vi "PicoCmdClientMove_5.vi"(1 "APulsesButton":bool, 2 "DeviceID":T1, 3 "Error in":errorcluster, 4 "ARateButton":bool, 5 "APulses":u16=300 step=100, 6 "Reverse":cluster{"Reverse X":bool, "Reverse Y":bool}, 7 "AXIS":u16(ring) items=["X", "Y or SLIDE", "Z"], 8 "aRate":dbl(ring)=1500.0 items=["375Hz"=375.0, "500Hz"=500.0, "750Hz"=750.0, "1500Hz"=1500.0], 9 "Move XY":T2(array[cluster]), 11 "aDir":bool=TRUE, 12 "connection ID in":refnum<k5>, 13 "aStop":bool, 16 "client name":string, 17 "Response?":bool) -> (20 "connection ID out":refnum<k5>, 21 "TCPconnectionCmd":bool, 25 "status":string, 27 "error out":errorcluster)   [LabVIEW 2013]
panel:
  out "Port":i32
  out "IPaddress":string
  out "mirror SlotConnector":i32
  out "Command":string
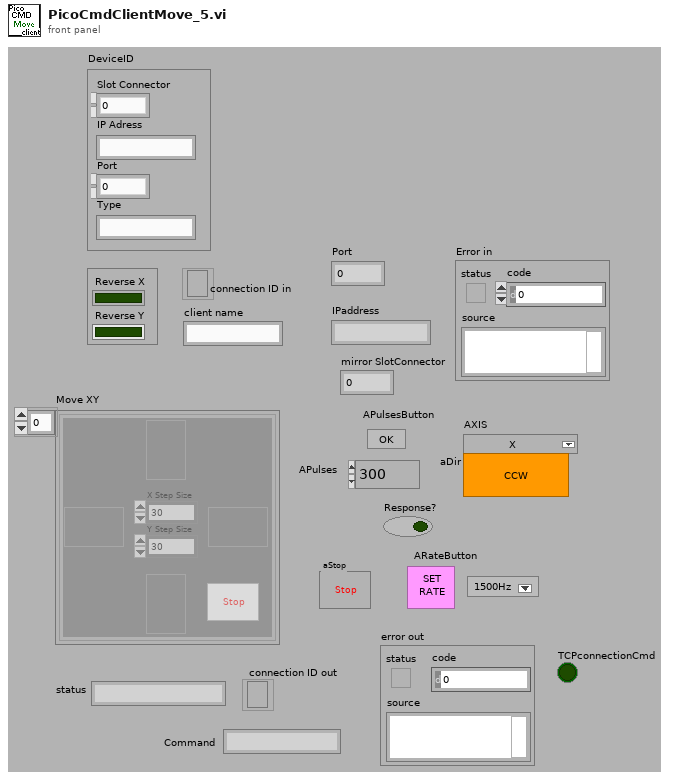
[diagram p1: front panel]
types:
  T1 = cluster{"Slot Connector":i32, "IP Adress":string, "Port":i32, "Type":string}
  T2 = cluster{"Down":bool, "Up":bool, "Right":bool, "Left":bool, "APulses X":u16, "APulses Y":u16, "Stop":bool}[]
  T3 = cluster{"Down":bool, "Up":bool, "Right":bool, "Left":bool, "APulses X":u16, "APulses Y":u16, "Left 2":bool}
  T4 = cluster{"Down":bool, "Up":bool, "Right":bool, "Left":bool, "APulses X":u16, "APulses Y":u16, "Left 2":bool}[]
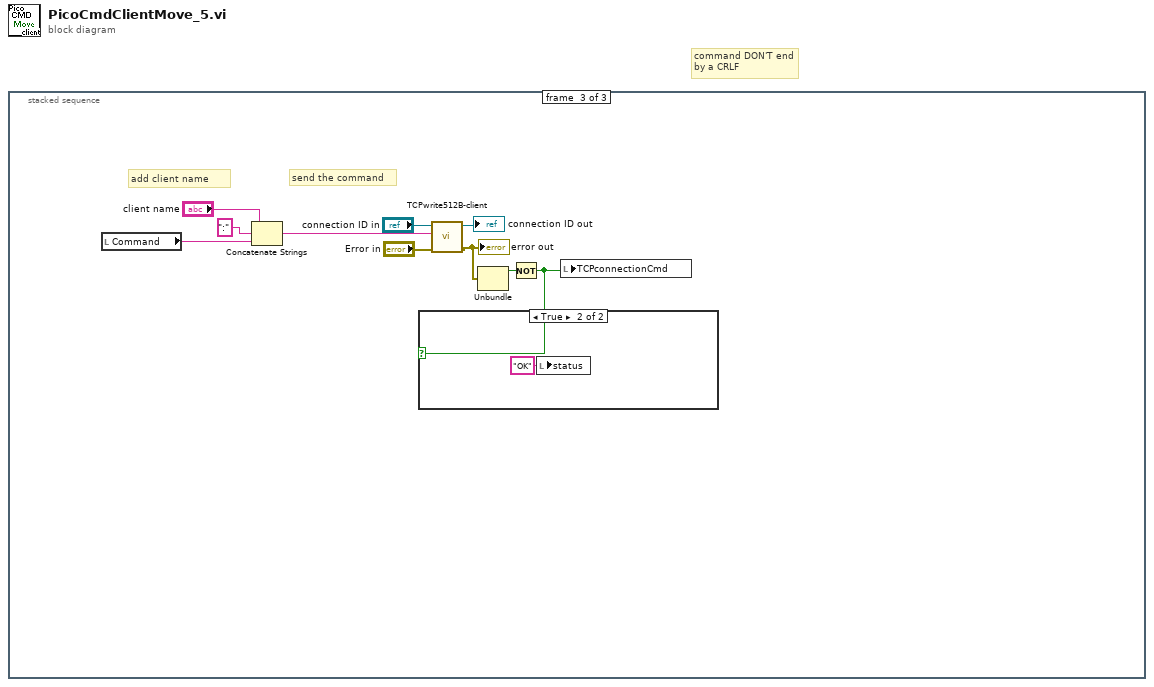
[diagram p0: block diagram]
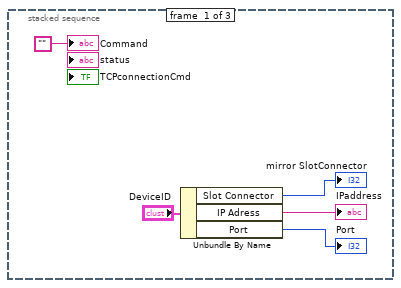
[diagram p2: hidden frame]
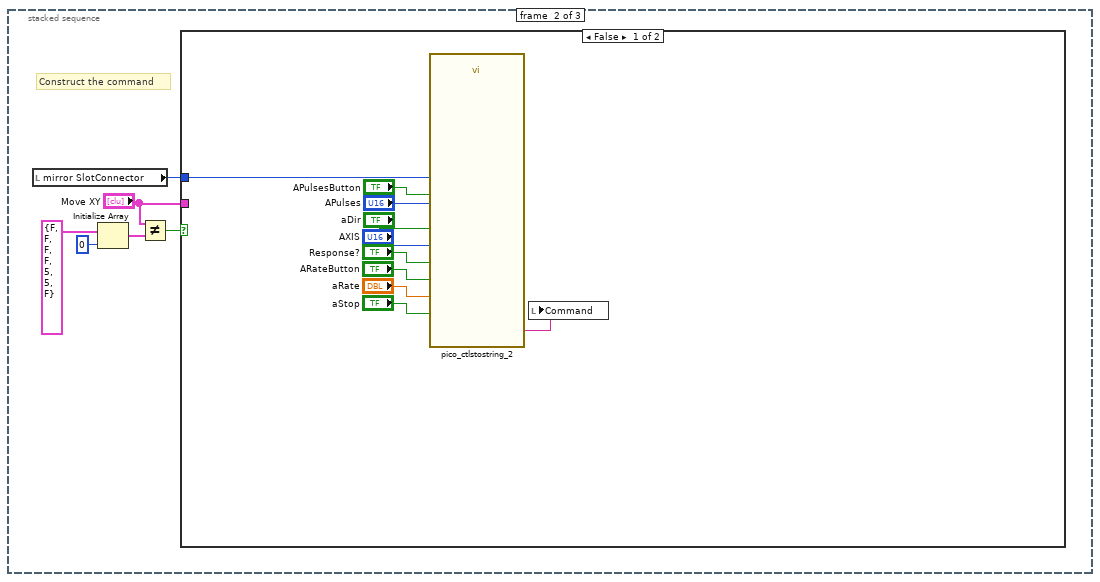
[diagram p3: hidden frame]
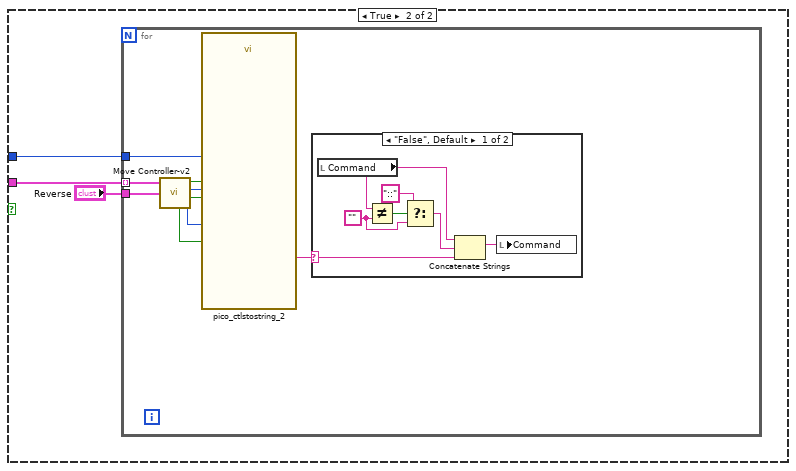
[diagram p4: hidden frame]
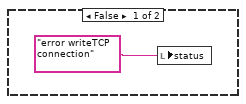
[diagram p6: hidden frame]
diagram:
  # "command DON'T end by a CRLF"
  n1 = stacked-sequence {
    frame #0 {
      n2 = Unbundle By Name("DeviceID") -> ("Slot Connector"=→"mirror SlotConnector":i32, "IP Adress"=→"IPaddress":string, "Port"=→"Port":i32)
      "Command" <- ""
    }
    frame #1 {
      # "Construct the command"
      n3 = local read "mirror SlotConnector"() -> (w6:i32)
      n4 = Initialize Array(T3 {"Down"=FALSE, "Up"=FALSE, "Right"=FALSE, "Left"=FALSE, "APulses X"=5, "APulses Y"=5, "Left 2"=FALSE} ("Corrective Move"), 0 ("dimension size")) -> (w11:T4)
      n5 = Not Equal?(x="Move XY", y=w11) -> (x != y?=w8:bool)
      n6 = case shown="False" w8 {
        tunnel: "Move XY" -> [_ w24]
        tunnel: w6 -> [w21 w23]
        frame False {
          n7 = call "pico_ctlstostring_2.vi"("Response?"="Response?", "AXIS"="AXIS", "MIRRORS"=w21, "aRate"="aRate", "ARateButton"="ARateButton", "aDir"="aDir", "aStop"="aStop", "APulses"="APulses", "APulsesButton"="APulsesButton") -> ("String out"=w12:string)
          n8 = local write "Command"(w12) -> ()
        }
        frame True {
          n9 = for {
            tunnel: w24 -> [w29] mode=indexing
            tunnel: w23 -> [w28]
            tunnel: "Reverse" -> [w25]
            n10 = call "Move Controller-v2.vi"("Move Control"=w29, "Reverse"=w25) -> ("Go"=w33:bool, "APulses"=w32:u16, "Direction"=w31:bool, "Axis (X=1,Y=2,Z=3)"=w30:u16, "Stop"=w26:bool)  [unwired: 1 in]
            n11 = call "pico_ctlstostring_2.vi"("AXIS"=w30, "MIRRORS"=w28, "aDir"=w31, "aStop"=w26, "APulses"=w32, "APulsesButton"=w33) -> ("String out"=w27:string)  [unwired: 3 in]
            n12 = case shown="\"False\", Default" w27 {
              selector: w27 -> [w34 _]
              frame "False", Default {
                w37 = ""
                n13 = local read "Command"() -> (w38:string)
                n14 = Not Equal?(x=w38, y=w37) -> (x != y?=w39:bool)
                n15 = Select(t="::" ("string"), s=w39, f=w37) -> (s? t:f=w35:string)
                n16 = Concatenate Strings(w38, w35, w34) -> (w40:string)
                n17 = local write "Command"(w40) -> ()
              }
              frame "" {
              }
            }
          }
        }
      }
    }
    frame #2 {
      # "send the command"
      # "add client name"
      n18 = local read "Command"() -> (w46:string)
      n19 = Concatenate Strings("client name", ":" ("string"), w46) -> (w42:string)
      n20 = call "TCPwrite512B-client.vi"("Error in"="Error in", "Cmd In"=w42, "connection ID in"="connection ID in") -> ("Error out"=w41:errorcluster, "connection ID out"=→"connection ID out":refnum<k5>)  [unwired: 7 out]
      "error out" <- w41
      n21 = Unbundle(w41) -> ("status"=w50:bool)  [unwired: 2 out]
      n22 = Not(x=w50) -> (.not. x?=w49:bool)
      n23 = case shown="True" w49 {
        frame False {
          n24 = local write "status"("error writeTCP connection" ("status")) -> ()
        }
        frame True {
          n25 = local write "status"("OK" ("status")) -> ()
        }
      }
      n26 = local write "TCPconnectionCmd"(w49) -> ()
    }
  }
